vi "messageClient.vi"() -> ()   [LabVIEW 2011]
panel:
  out "error out":errorcluster
  in  "queueName":string="messageQue"
  in  "OK Button":bool
  in  "port":u16
  in  "ip":string="127.0.0.1"
  out "MessageLog":string[](array[string])
  in  "data in":string="0002ab"
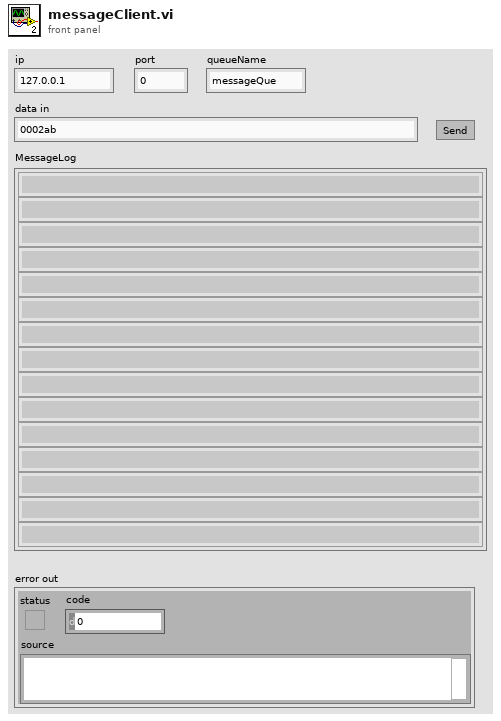
[diagram p1: front panel]
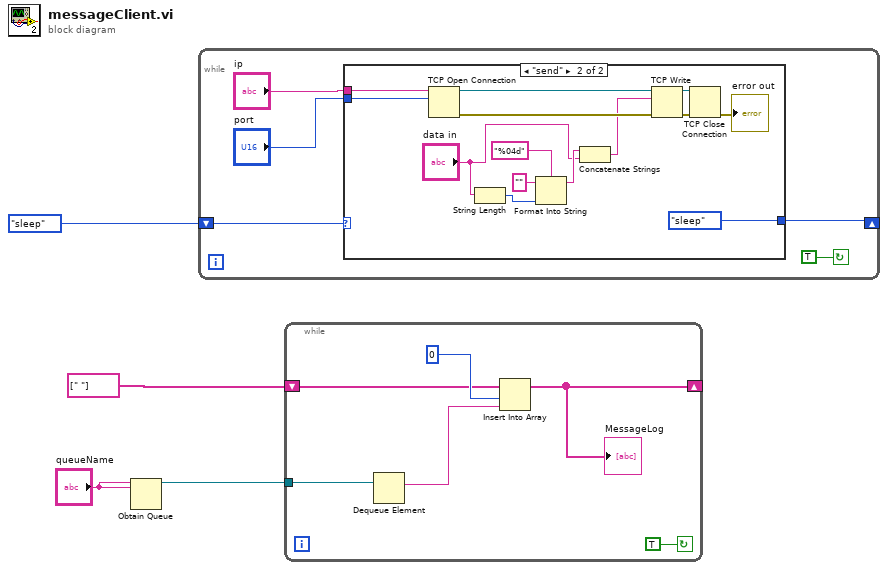
[diagram p0: block diagram]
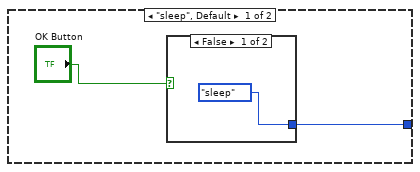
[diagram p2: hidden frame]
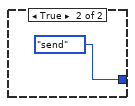
[diagram p3: hidden frame]
diagram:
  n1 = Obtain Queue(name (unnamed)="queueName", element data type="queueName") -> (queue out=w3:refnum<queue>)  [unwired: 3 in, 2 out]
  n2 = while {
    shift-right: [w7] -> _
    shift-left: enum16{"sleep", "send"}."sleep" ("Enum") -> [w8]
    stop <- TRUE continue-if-true
    n3 = case shown="\"send\"" w8 {
      tunnel: "ip" -> [_ w27]
      tunnel: "port" -> [_ w26]
      tunnel: [w10 enum16{"sleep", "send"}."sleep" ("Enum")] -> w7
      frame "sleep", Default {
        n4 = case shown="False" "OK Button" {
          tunnel: [enum16{"sleep", "send"}."sleep" ("Enum") enum16{"sleep", "send"}."send" ("Enum")] -> w10
          frame False {
          }
          frame True {
          }
        }
      }
      frame "send" {
        n5 = TCP Open Connection(address=w27, remote port or service name=w26) -> (connection ID=w25:refnum<k5>, error out=w24:errorcluster)  [unwired: 3 in]
        n6 = String Length(string="data in") -> (length=w21:i32)
        n7 = Format Into String(format string="%04d", initial string="", w21) -> (resulting string=w19:string)  [unwired: 1 in, 1 out]
        n8 = Concatenate Strings(w19, "data in") -> (w17:string)
        n9 = TCP Write(connection ID=w25, data in=w17, error in (no error)=w24) -> (connection ID out=w22:refnum<k5>, error out=w23:errorcluster)  [unwired: 1 in, 1 out]
        n10 = TCP Close Connection(connection ID=w22, error in (no error)=w23) -> (error out=→"error out":errorcluster)  [unwired: 1 in, 1 out]
      }
    }
  }
  n11 = while {
    tunnel: w3 -> [w33]
    shift-right: [w28] -> _
    shift-left: string[] [" "] ("Array") -> [w30]
    stop <- TRUE continue-if-true
    n12 = Dequeue Element(queue=w33) -> (element=w31:string)  [unwired: 2 in, 3 out]
    n13 = Insert Into Array(array=w30, index=0, new element=w31) -> (w28:string[])
    "MessageLog" <- w28
  }
